vi "corrupt_Connect Channels.vi"(8 "error in (no error)":errorcluster, 11 "CIFTemplateNode in":refnum<class "CIFCorePlugin.lvclass">) -> (0 "error out":errorcluster, 3 "CIFTemplateNode out":refnum<class "CIFCorePlugin.lvclass">)   [LabVIEW 2021]
uses:
  CIFCorePlugin.lvclass
  CIFCorePlugin.lvclass/CIFCorePlugin.ctl
  CIFUtilities/CIFOutOfBand/CIFOutOfBand.lvclass/CIFOutOfBand.ctl
  OOB/OOB_Rx/CIFCoreOOB_Rx.lvclass/CIFCoreOOB_Rx.ctl
  Channels/CIFChannelMng/CIFChannelMng.lvclass/CIFChannelMng.ctl
  Channels/CIFChannels/CIFChannels.lvclass/CIFChannels.ctl
  OOB/OOB_Rx/Private/Read Payload.vi
  Channels/CIFChannelMng/Utilities/Get Channel Index by Name.vi
  Channels/CIFChannels/Accessors/Read Channel State.vi
  CIFUtilities/CIFOutOfBand/Accessors/Read Local OOB Data.vi
  CIFUtilities/CIFClocks/SubVIs/Add Error.vi
  Common/Utilities/Append Error Location.vi
  OOB/OOB_Rx/CIFCoreOOB_Rx.lvclass
  D:/dev/CIF-LVCore/src/CIFUtilities/CIFOutOfBand/CIFOutOfBand.lvclass
  Channels/CIFChannels/CIFChannels.lvclass
  Channels/CIFChannelMng/CIFChannelMng.lvclass
  D:/dev/CIF-LVCore/src/CIFCore/OOB/OOB_Rx/CIFCoreOOB_Rx.lvclass
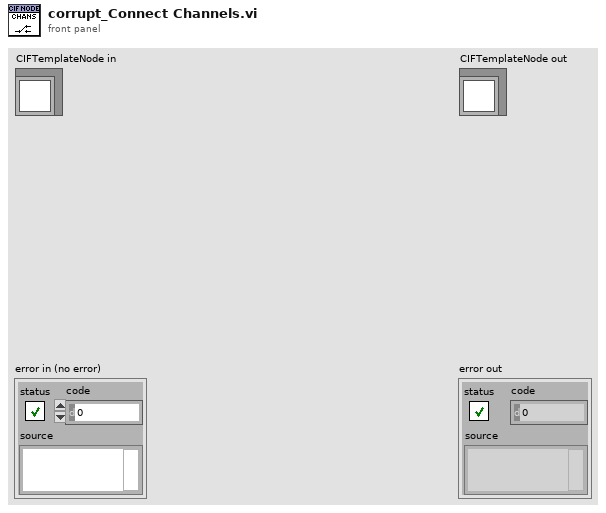
[diagram p1: front panel]
types:
  T1 = typedef "CIFCoreOOB_Rx.lvclass/Channel Connection Data.ctl" = cluster{"Publisher Name":string, "Subscriber Name":string, "Connection Data":u8[]}
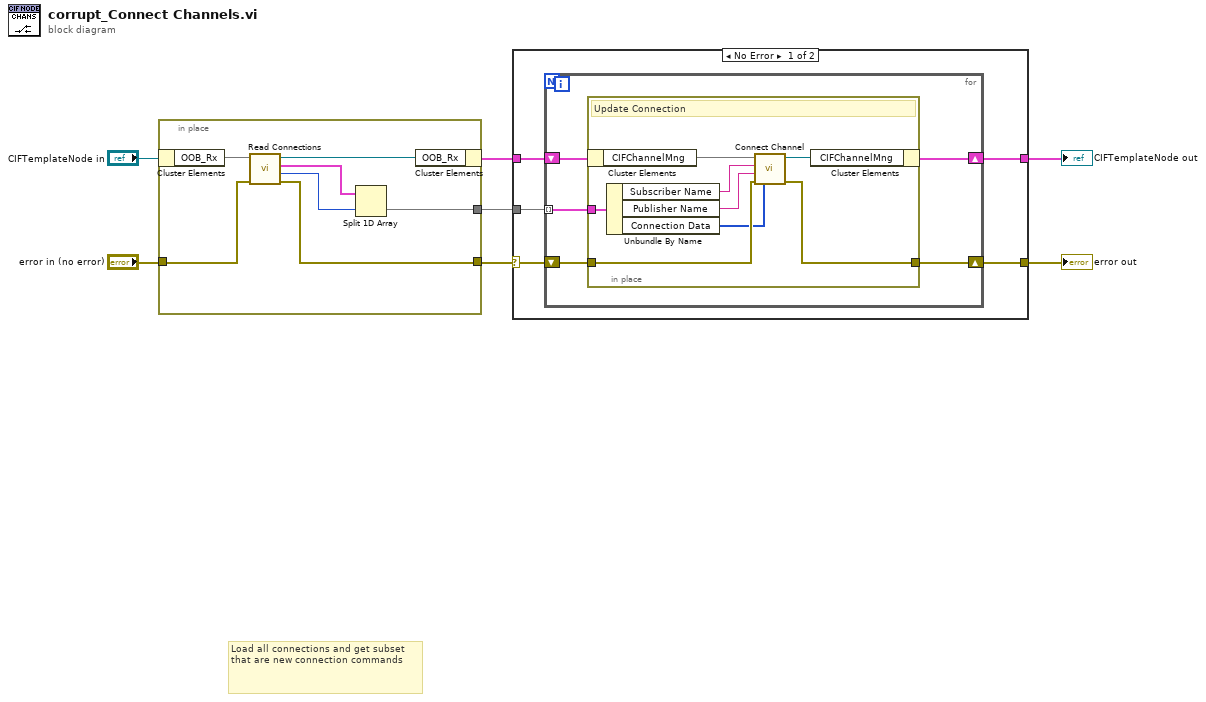
[diagram p0: block diagram]
diagram:
  # "Load all connections and get subset that are new connection commands"
  n1 = in-place {
    in-place-border: "error in (no error)" -> [w13]
    in-place-border: [w11] -> w4
    in-place-border: [w8] -> w3
    n2 = in-place-cluster #1("CIFTemplateNode in") -> ("OOB_Rx"=w14)
    n3 = call "Read Connections.vi"("error in"=w13, "CoreOOB_Rx in"=w14) -> ("error out"=w11:errorcluster, "Offset"=w10:i32, "Connections"=w9:T1[], "CoreOOB_Rx out"=w12:refnum<class "CIFCoreOOB_Rx.lvclass">)  [unwired: 6 in]
    n4 = Split 1D Array(array=w9, index=w10) -> (second subarray=w8:T1[])  [unwired: 1 out]
    n5 = in-place-cluster #1("OOB_Rx"=w12) -> (w5:cluster{})
  }
  n6 = case shown="No Error" w4 {
    selector: w4 -> [w17 w33]
    tunnel: w5 -> [w18 w34]
    tunnel: w3 -> [w19 _]
    tunnel: [w16 w33] -> w2
    tunnel: [w15 w34] -> w1
    frame No Error {
      n7 = for {
        tunnel: w19 -> [w23] mode=indexing
        shift-right: [w20] -> w15
        shift-left: w18 -> [w24]
        shift-right: [w21] -> w16
        shift-left: w17 -> [w22]
        n8 = in-place {
          in-place-border: w23 -> [w31]
          in-place-border: w22 -> [w30]
          in-place-border: [w25] -> w21
          # "Update Connection"
          n9 = in-place-cluster #2(w24) -> ("CIFChannelMng"=w32)
          n10 = Unbundle By Name(w31) -> ("Subscriber Name"=w28:string, "Publisher Name"=w27:string, "Connection Data"=w29:u8[])
          n11 = call "Connect Channel.vi"("Custom Channel Config Data"=w29, "error in (no error)"=w30, "Publisher Name"=w27, "Subscriber Name"=w28, "CIFChannelMng in"=w32) -> ("error out"=w25:errorcluster, "CIFChannelMng out"=w26:refnum<class "CIFChannelMng.lvclass">)  [unwired: 5 in]
          n12 = in-place-cluster #2("CIFChannelMng"=w26) -> (w20:cluster{})
        }
      }
    }
    frame Error {
    }
  }
  "error out" <- w2
  "CIFTemplateNode out" <- w1
